vi "Ini key write (DBL).vi"(7 "Section":string, 8 "error in (no error)":errorcluster, 9 "Values (DBL)":dbl[](array[numeric]), 10 "Ini file interface":T2, 11 "Ini file refnum in":T1) -> (0 "error out":errorcluster, 3 "Ini file refnum out":T1)   [LabVIEW 2017]
uses:
  <vilib>/Utility/config.llb/Config Data RefNum.ctl
  Typedefs/Ini file interface (DBL).ctl
  <vilib>/Utility/config.llb/Write Key (Double).vi
  <vilib>/Utility/config.llb/Read Key (Double).vi
  <vilib>/Utility/config.llb/NI_LVConfig.lvlib
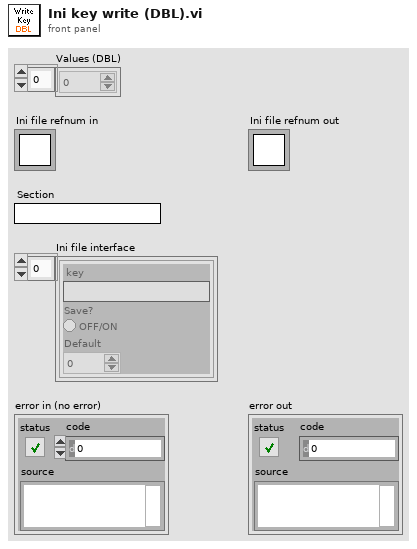
[diagram p1: front panel]
types:
  T1 = typedef "NI_LVConfig.lvlib/Config Data RefNum.ctl" = refnum<k1>
  T2 = typedef "Ini file interface (DBL).ctl" = cluster{"key":string, "Save?":bool, "Default":dbl}[]
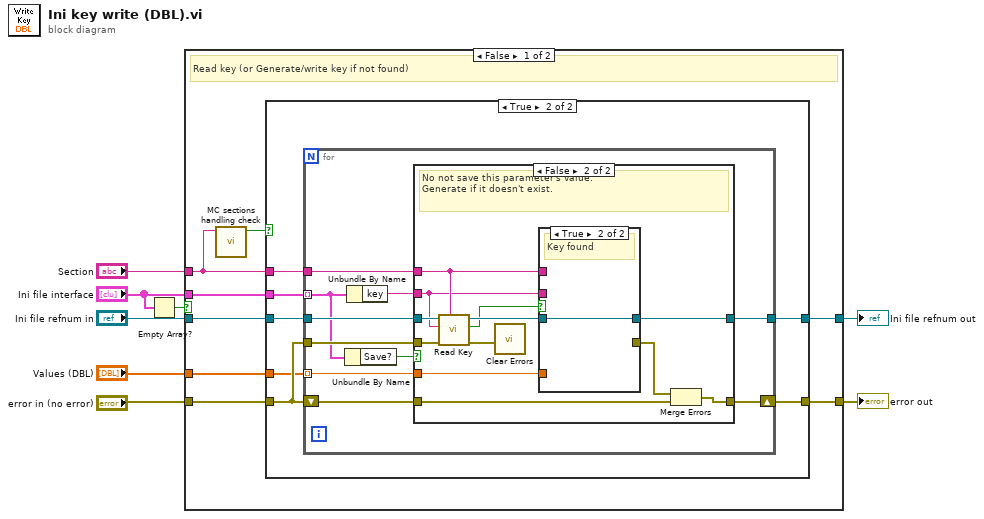
[diagram p0: block diagram]
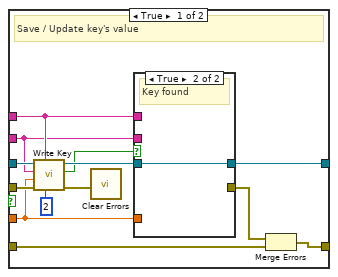
[diagram p3: hidden frame]
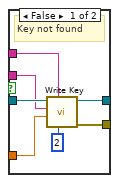
[diagram p4: hidden frame]
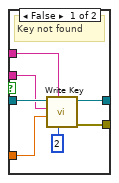
[diagram p5: hidden frame]
diagram:
  n1 = Empty Array?(array="Ini file interface") -> (empty?=w3:bool)
  n2 = case shown="False" w3 {
    tunnel: "Ini file refnum in" -> [w16 w78]
    tunnel: [w15 w78] -> w8
    tunnel: [w14 w77] -> w7
    tunnel: "error in (no error)" -> [w13 w77]
    tunnel: "Section" -> [w10 _]
    tunnel: "Ini file interface" -> [w12 _]
    tunnel: "Values (DBL)" -> [w11 _]
    frame False {
      # "Read key (or Generate/write key if not found)"
      n3 = call "MC sections handling check.vi"("Section name"=w10) -> ("Section is \"Initial MovCor Values\" AND MC is supported"=w9:bool)  [unwired: 10 in]
      n4 = case shown="True" w9 {
        tunnel: w16 -> [w18 w25]
        tunnel: [w18 w24] -> w15
        tunnel: [w17 w23] -> w14
        tunnel: w13 -> [w17 w22]
        tunnel: w12 -> [_ w21]
        tunnel: w11 -> [_ w20]
        tunnel: w10 -> [_ w19]
        frame False {
          # "The [Initial MovCor Values] section not handled when the MC UI is unavailable"
        }
        frame True {
          n5 = for {
            tunnel: w25 -> [w35]
            tunnel: w22 -> [w34]
            tunnel: [w33] -> w24
            shift-right: [w32] -> w23
            shift-left: w22 -> [w31]
            tunnel: w21 -> [w27] mode=indexing
            tunnel: w20 -> [w30] mode=indexing
            tunnel: w19 -> [w29]
            n6 = Unbundle By Name(w27) -> ("Save?"=w26:bool)
            n7 = Unbundle By Name(w27) -> ("key"=w28:string)
            n8 = case shown="False" w26 {
              tunnel: w35 -> [w48 w68]
              tunnel: w34 -> [w47 w67]
              tunnel: [w38 w58] -> w33
              tunnel: [w46 w66] -> w32
              tunnel: w31 -> [w45 w65]
              tunnel: w28 -> [w41 w61]
              tunnel: w30 -> [w39 w59]
              tunnel: w29 -> [w42 w62]
              frame True {
                # "Save / Update key's value"
                n9 = call-poly <vilib>:"Write Key.vi"("precision (6)"=i16 2, "section"=w42, "error in (no error)"=w47, "value"=w39, "key"=w41, "refnum"=w48) -> ("error out"=w44:errorcluster, "found?"=w37:bool, "refnum out"=w43:T1)  [unwired: 3 in]
                n10 = call <vilib>:"Clear Errors.vi"("error in (no error)"=w44) -> ()  [unwired: 5 in, 2 out]
                n11 = case shown="True" w37 {
                  tunnel: w43 -> [w55 w56]
                  tunnel: [w54 w56] -> w38
                  tunnel: [w53 _] -> w40
                  tunnel: w42 -> [w52 _]
                  tunnel: w41 -> [w51 _]
                  tunnel: w39 -> [w50 _]
                  frame False {
                    # "Key not found"
                    n12 = call-poly <vilib>:"Write Key.vi"("precision (6)"=i16 2, "section"=w52, "value"=w50, "key"=w51, "refnum"=w55) -> ("error out"=w53:errorcluster, "refnum out"=w54:T1)  [unwired: 4 in, 1 out]
                  }
                  frame True {
                    # "Key found"
                  }
                }
                n13 = Merge Errors(w40, w45) -> (w46:errorcluster)
              }
              frame False {
                # "No not save this parameter's value.\nGenerate if it doesn't exist."
                n14 = call-poly <vilib>:"Read Key.vi"("section"=w62, "error in (no error)"=w67, "key"=w61, "refnum"=w68) -> ("error out"=w64:errorcluster, "found?"=w57:bool, "refnum out"=w63:T1)  [unwired: 4 in, 1 out]
                n15 = call <vilib>:"Clear Errors.vi"("error in (no error)"=w64) -> ()  [unwired: 5 in, 2 out]
                n16 = case shown="True" w57 {
                  tunnel: w63 -> [w75 w76]
                  tunnel: [w74 w76] -> w58
                  tunnel: [w73 _] -> w60
                  tunnel: w62 -> [w72 _]
                  tunnel: w61 -> [w71 _]
                  tunnel: w59 -> [w70 _]
                  frame False {
                    # "Key not found"
                    n17 = call-poly <vilib>:"Write Key.vi"("precision (6)"=i16 2, "section"=w72, "value"=w70, "key"=w71, "refnum"=w75) -> ("error out"=w73:errorcluster, "refnum out"=w74:T1)  [unwired: 4 in, 1 out]
                  }
                  frame True {
                    # "Key found"
                  }
                }
                n18 = Merge Errors(w60, w65) -> (w66:errorcluster)
              }
            }
          }
        }
      }
    }
    frame True {
      # "Setup array is empty"
    }
  }
  "Ini file refnum out" <- w8
  "error out" <- w7
